vi "HGF_TimeoutWorker.appendData2Variant.vi"(0 "initData":variant, 2 "timeout(ms)":i32, 5 "error in":errorcluster) -> (14 "initData":variant, 19 "error out":errorcluster)   [LabVIEW 2014, in "HGF_BaseClasses.lvlib" / "HGF_TimeoutWorker.lvclass"]
uses:
  HGF_TimeoutWorker.lvclass
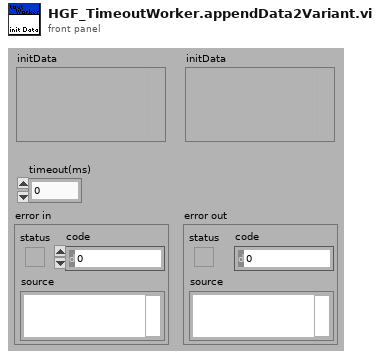
[diagram p1: front panel]
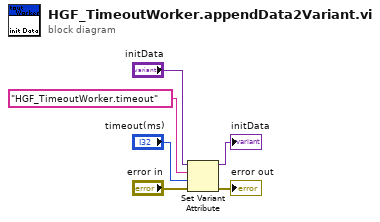
[diagram p0: block diagram]
diagram:
  n1 = Set Variant Attribute(Variant="initData", name="HGF_TimeoutWorker.timeout", value="timeout(ms)", error in="error in") -> (Variant out=→"initData":variant, error out=→"error out":errorcluster)  [unwired: 1 out]
